vi "SECoP-createNode.vi"(7 "description":string, 8 "error in (no error)":errorcluster, 9 "TCP port":u16=2055, 10 "node id":string, 11 "DLL path (in)":T1) -> (0 "error out":errorcluster, 3 "DLL path (out)":T1)   [LabVIEW 2023, in "SECoP.lvlib"]
doc: "Call <b>\"SECoP-createNode.vi\"</b> to create an empty SECoP node. You need at least one for a working SEC-node. Every node exists independent of each other, but it is up to the user, how they act.\n\n<b>DLL path</b> input and output of cluster from \"SECoP-Initialize.vi\"\n<b>node id</b> unique name of the SECoP node\n<b>description</b> a mandatory description text\n<b>TCP port</b> port to listen to"
uses:
  SECoP.lvlib
  SECoP-libraries.ctl
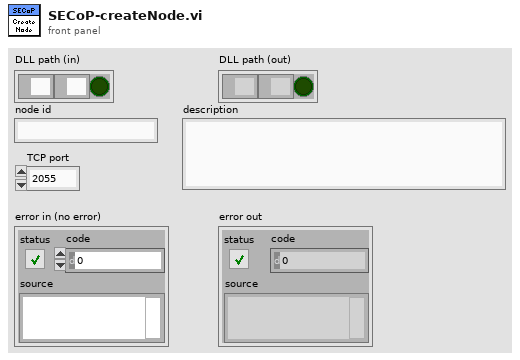
[diagram p1: front panel]
types:
  T1 = typedef "SECoP.lvlib/SECoP-libraries.ctl" = cluster{"serverDLL":path, "variantDLL":path, "cleanup_mode":bool}
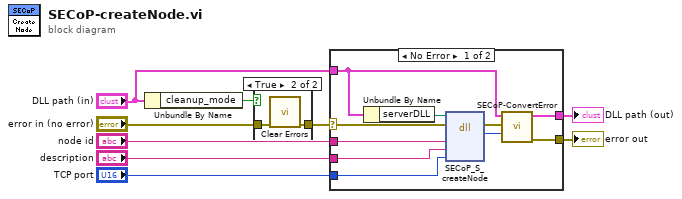
[diagram p0: block diagram]
diagram:
  n1 = Unbundle By Name("DLL path (in)") -> ("cleanup_mode"=w4:bool)
  n2 = case shown="True" w4 {
    tunnel: "error in (no error)" -> [w10 w12]
    tunnel: [w10 w11] -> w2
    frame False {
    }
    frame True {
      n3 = call <vilib>:"Clear Errors.vi"("error in (no error)"=w12) -> ("error out"=w11:errorcluster)  [unwired: 5 in, 1 out]
    }
  }
  n4 = case shown="No Error" w2 {
    selector: w2 -> [w20 w23]
    tunnel: "DLL path (in)" -> [w14 w24]
    tunnel: [w21 w24] -> w9
    tunnel: [w22 w23] -> w8
    tunnel: "node id" -> [w17 _]
    tunnel: "description" -> [w16 _]
    tunnel: "TCP port" -> [w15 _]
    frame No Error {
      n5 = Unbundle By Name(w14) -> ("serverDLL"=w13:path)
      n6 = dll-call lib="C:/Users/user/Desktop/x86_64/SECoP64.dll" fn="SECoP_S_createNode"(path in=w13, error in=w20, "id"=w17, "description"=w16, "TCP port"=w15) -> (error out=w19:errorcluster, "return type"=w18:i32)  [unwired: 4 in, 1 out]
      n7 = call "SECoP-ConvertError.vi"("return code"=w18, "error in (no error)"=w19, "DLL path (in)"=w14) -> ("error out"=w22:errorcluster, "DLL path (out)"=w21:T1)  [unwired: 7 in]
    }
    frame Error {
    }
  }
  "DLL path (out)" <- w9
  "error out" <- w8
